vi "DEMO_01_SER_PRO.vi"() -> ()   [LabVIEW 2014]
uses:
  <vilib>/Instr/_visa.llb/VISA Configure Serial Port (Instr).vi
panel:
  out "输出变量":dbl
  in  "读取数据":bool
  in  "数据值":dbl
  in  "发送":bool
  in  "开闭环":u16(ring) items=["  开环", "  闭环"]
  in  "打开串口":bool
  in  "上位机控制":bool
  in  "波特率":u32(ring)=9600 items=["75"=75, "110"=110, "134"=134, "150"=150, "300"=300, "600"=600, "1200"=1200, "1800"=1800, "2400"=2400, "4800"=4800, "7200"=7200, "9600"=9600, "14400"=14400, "19200"=19200, "28800"=28800, "38400"=38400, "56000"=56000, "57600"=57600, "115200"=115200, "128000"=128000, "230400"=230400]
  in  "奇偶":enum16{"None", "Odd", "Even", "Mark", "Space"}(ring) caption="校验"
  in  "VISA资源名称":refnum<visa-resource-name>="COM1"
  in  "通道选择":u16(ring) items=["一路", "二路", "三路"]
  # "单点数据控制"
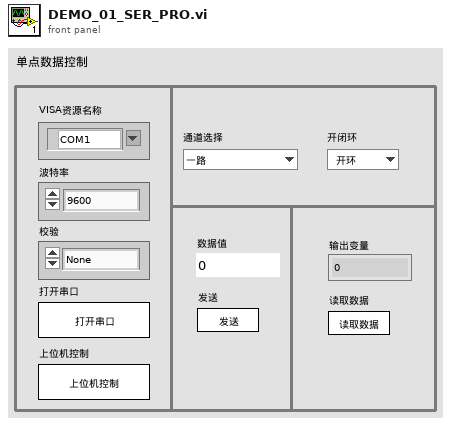
[diagram p1: front panel]
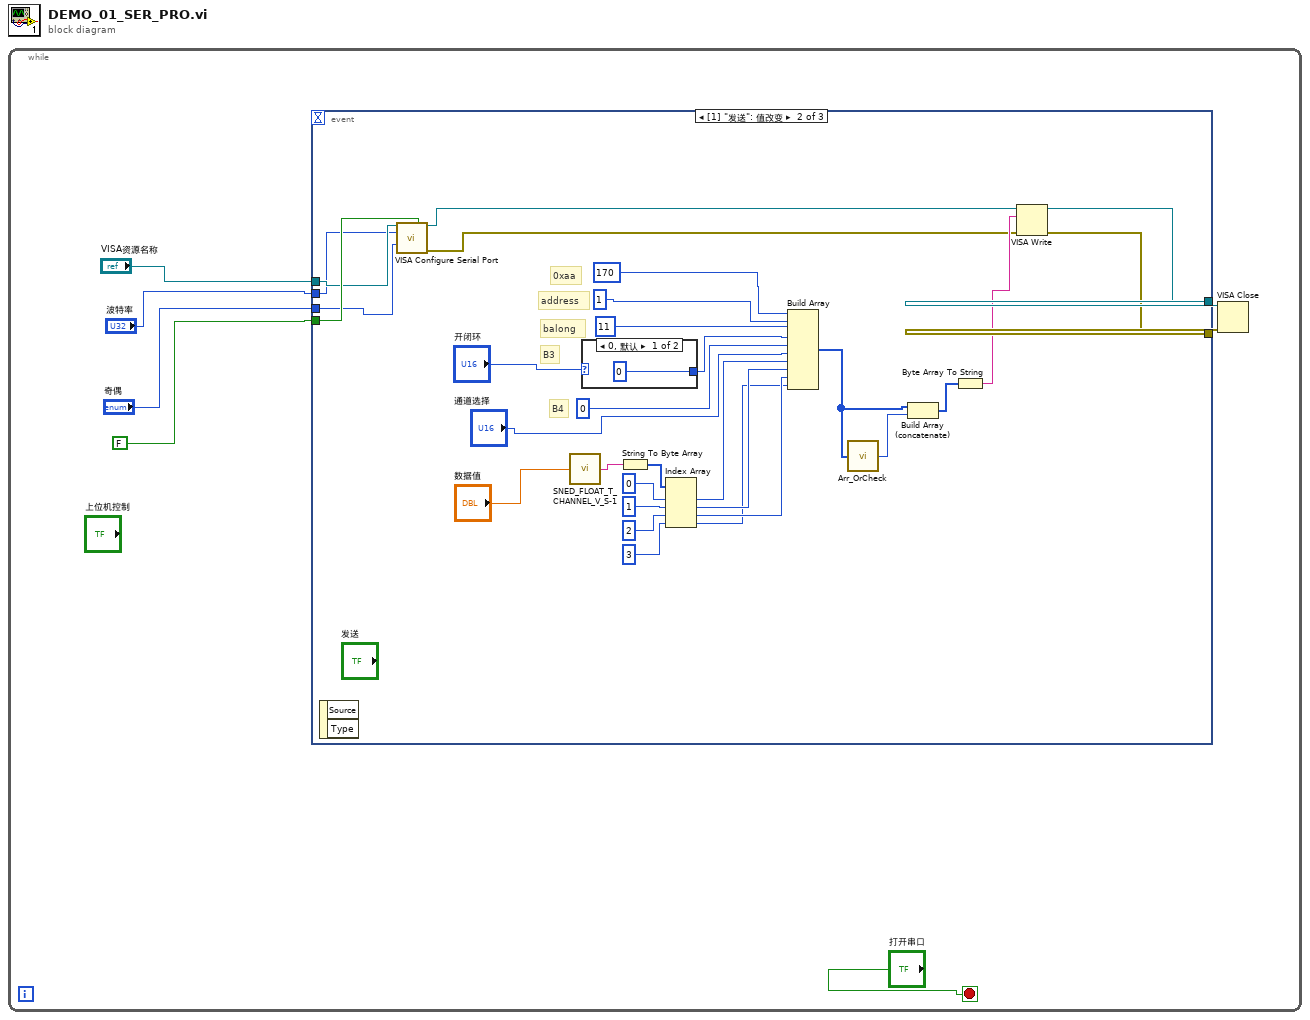
[diagram p0: block diagram]
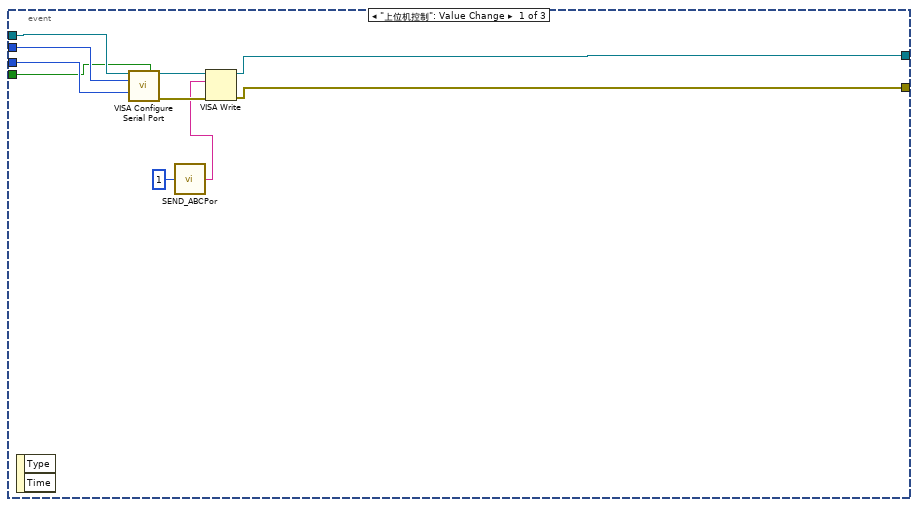
[diagram p2: hidden frame]
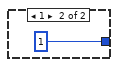
[diagram p3: hidden frame]
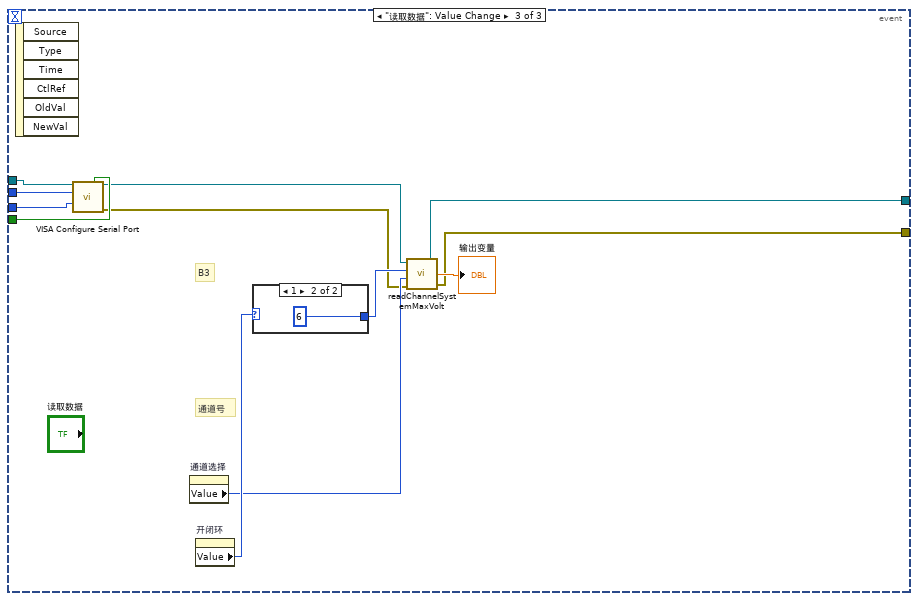
[diagram p4: hidden frame]
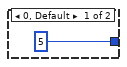
[diagram p5: hidden frame]
diagram:
  n1 = while {
    stop <- "打开串口" stop-if-true
    n2 = event shown="[1] \"发送\": 值改变" {
      selector: _ -> [_ _ _]
      dyn-events: _ -> [_ _ _]
      timeout: _ -> [_ _ _]
      tunnel: [w17 w33 w50] -> w6
      tunnel: [w16 w32 w57] -> w5
      tunnel: FALSE -> [w10 w47 w61]
      tunnel: "VISA资源名称" -> [w13 w45 w60]
      tunnel: "波特率" -> [w12 w44 w59]
      tunnel: "奇偶" -> [w11 w46 w58]
      event "上位机控制": Value Change {
        n3 = event-data() -> ()  [unwired: 1 in, 2 out]
        n4 = call-poly "VISA Configure Serial Port"("VISA resource name"=w13, "Enable Termination\nChar (T)"=w10, "baud rate (9600)"=w12, "parity (0:none)"=w11) -> ("VISA resource name out"=w15:refnum<visa-resource-name>, "error out"=w14:errorcluster)  [unwired: 10 in]
        n5 = call "SEND_ABCPor.vi"("设备地址 1 开始"=1) -> ("输出字符串"=w8:string)
        n6 = VISA Write(VISA resource name=w15, write buffer=w8, error in (no error)=w14) -> (VISA resource name out=w16:refnum<visa-resource-name>, error out=w17:errorcluster)  [unwired: 1 out]
      }
      event "发送": Value Change {
        # "B4"
        # "B3"
        # "balong"
        # "address"
        # "0xaa"
        n7 = event-data() -> ()  [unwired: 1 in, 2 out]
        n8 = call-poly "VISA Configure Serial Port"("VISA resource name"=w45, "Enable Termination\nChar (T)"=w47, "baud rate (9600)"=w44, "parity (0:none)"=w46) -> ("VISA resource name out"=w34:refnum<visa-resource-name>, "error out"=w20:errorcluster)  [unwired: 10 in]
        n9 = call "SNED_FLOAT_T_CHANNEL_V_S-1.vi"("数据"="数据值") -> ("字符串"=w43:string)
        n10 = case shown="0, 默认" "开闭环" {
          tunnel: [0 1] -> w27
          frame 0, Default {
          }
          frame 1 {
          }
        }
        n11 = String To Byte Array(string=w43) -> (unsigned byte array=w42:u8[])
        n12 = Index Array(array=w42, index #1=0, index #2=1, index #3=2, index #4=3) -> (element #1=w25:u8, element #2=w24:u8, element #3=w23:u8, element #4=w22:u8)
        n13 = Build Array(170, 1, 11, w27, 0, "通道选择", w25, w24, w23, w22) -> (w21:i32[])
        n14 = call "Arr_OrCheck.vi"("数组"=w21) -> ("抑或的数据值"=w37:u8)
        n15 = Build Array (concatenate)(w21, w37) -> (w36:i32[])
        n16 = Byte Array To String(unsigned byte array=w36) -> (string=w35:string)
        n17 = VISA Write(VISA resource name=w34, write buffer=w35, error in (no error)=w20) -> (VISA resource name out=w32:refnum<visa-resource-name>, error out=w33:errorcluster)  [unwired: 1 out]
      }
      event "读取数据": Value Change {
        # "通道号"
        # "B3"
        n18 = event-data() -> ()  [unwired: 1 in, 6 out]
        n19 = call-poly "VISA Configure Serial Port"("VISA resource name"=w60, "Enable Termination\nChar (T)"=w61, "baud rate (9600)"=w59, "parity (0:none)"=w58) -> ("VISA resource name out"=w53:refnum<visa-resource-name>, "error out"=w51:errorcluster)  [unwired: 10 in]
        n20 = property on="通道选择" class="Ring (严格)"() -> ("Value"=w55:u16)  [unwired: 2 in, 2 out]
        n21 = property on="开闭环" class="Ring (严格)"() -> ("Value"=w56:u16)  [unwired: 2 in, 2 out]
        n22 = case shown="1" w56 {
          tunnel: [5 6] -> w54
          frame 0, Default {
          }
          frame 1 {
          }
        }
        n23 = call "readChannelSystemMaxVolt.vi"("error out 2"=w51, "通道号"=w55, "B3"=w54, "VISA resource name out 2"=w53) -> ("error out"=w50:errorcluster, "输出变量"=→"输出变量":dbl, "VISA resource name out"=w57:refnum<visa-resource-name>)
      }
    }
    n24 = VISA Close(VISA resource name=w5, error in (no error)=w6) -> ()  [unwired: 1 out]
  }
